vi "Move.vi"(8 "error in (no error)":errorcluster, 9 "type":enum16{"Rapid (G0)", "Linear (G1)"}(ring)=enum."Linear (G1)", 10 "Distances":T1, 11 "VISA resource name":refnum<visa-resource-name>) -> (0 "error out":errorcluster, 3 "VISA resource name out":refnum<visa-resource-name>)   [LabVIEW 2020, in "Marlin Instrument Driver.lvlib"]
doc: "Returns the current state of the configured X, Y, Z endstops. Takes into account any 'inverted endstop' settings, so one can confirm that the machine is interpreting the endstops correctly."
uses:
  <instrlib>/Marlin Instrument Driver/Marlin Instrument Driver.lvlib
  <instrlib>/Marlin Instrument Driver/Public/controls/move parameters.ctl
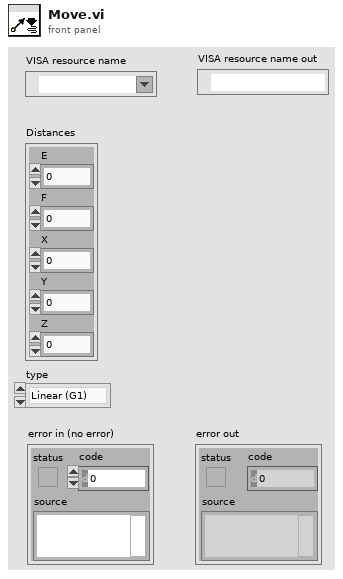
[diagram p1: front panel]
types:
  T1 = typedef "Marlin Instrument Driver.lvlib/move parameters.ctl" = cluster{"E":dbl, "F":dbl, "X":dbl, "Y":dbl, "Z":dbl}
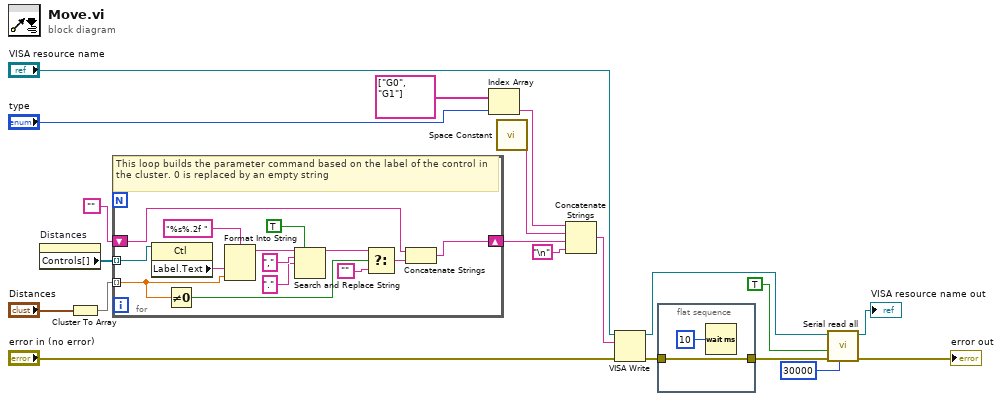
[diagram p0: block diagram]
diagram:
  n1 = property on="Distances" class="Clust (strict)"() -> ("Controls[]"=w11:refnum<vi>[])  [unwired: 2 in, 2 out]
  n2 = Cluster To Array(cluster="Distances") -> (array=w12:dbl[])
  n3 = for {
    tunnel: w12 -> [w29] mode=indexing
    tunnel: w11 -> [w34] mode=indexing
    shift-right: [w31] -> w5
    shift-left: "" -> [w32]
    # "This loop builds the parameter command based on the label of the control in the cluster. 0 is replaced by an empty string"
    n4 = property class="Ctl"(reference=w34) -> ("Label.Text"=w33:string)  [unwired: 1 in, 2 out]
    n5 = Not Equal To 0?(x=w29) -> (x != 0?=w28:bool)
    n6 = Format Into String(format string="%s%.2f ", w33, w29) -> (resulting string=w25:string)  [unwired: 2 in, 1 out]
    n7 = Search and Replace String(replace all?=TRUE ("replace all? (F)"), input string=w25, search string=",", replace string="." ("replace string (\"\")")) -> (result string=w24:string)  [unwired: 4 in, 3 out]
    n8 = Select(t=w24, s=w28, f="") -> (s? t:f=w27:string)
    n9 = Concatenate Strings(w32, w27) -> (w31:string)
  }
  n10 = Index Array(array=string[] ["G0", "G1"], index="type") -> (element=w8:string)
  n11 = call <vilib>:"Space Constant.vi"() -> ("String"=w6:string)
  n12 = Concatenate Strings(w8, w6, w5, "\n") -> (w3:string)
  n13 = VISA Write(VISA resource name="VISA resource name", write buffer=w3, error in (no error)="error in (no error)") -> (VISA resource name out=w18:refnum<visa-resource-name>, error out=w2:errorcluster)  [unwired: 1 out]
  n14 = flat-sequence {
    tunnel: [w35] -> w1
    tunnel: w2 -> [w35]
    frame #0 {
      n15 = Wait (ms)(milliseconds to wait=u32 10) -> ()  [unwired: 1 out]
    }
  }
  n16 = call <instrlib>:"Serial read all.vi"("timeout (10000ms)"=u32 30000, "error in (no error)"=w1, "Wait for OK"=TRUE, "VISA Refnum in"=w18) -> ("error out"=→"error out":errorcluster, "VISA Refnum out"=→"VISA resource name out":refnum<visa-resource-name>)  [unwired: 4 in, 2 out]
